vi "Remove Waveforms from ListBox.vi"(5 "Names List":bool, 7 "UI Refs":T2, 8 "error in":errorcluster, 9 "Waveform Ref LUT":variant, 10 "CD Settings in":T3 {"CD Task Dependency Ref" format="%.0x"; "CD Task Dependency" format="%.0x"}, 11 "Custom Device Ref in":T1 format="%.0x") -> (0 "error out":errorcluster, 1 "Waveform Ref LUT out":variant, 2 "CD Settings out":T3 {"CD Task Dependency Ref" format="%.0x"; "CD Task Dependency" format="%.0x"}, 3 "Custom Device Ref out":T1 format="%.0x")   [LabVIEW 2017, in "Waveform-Processing-Custom-Device System Explorer.lvlib"]
uses:
  Waveform-Processing-Custom-Device System Explorer.lvlib
  Shared/Custom Device Settings.ctl
  <vilib>/NI Veristand/Custom Device API/Custom Device Item Ref.ctl
  Types/UI Refs Ctl.ctl
  <vilib>/NI Veristand/Custom Device API/Custom Device Pointer.ctl
  NationalInstruments.VeriStand.SystemStorage
  NationalInstruments.VeriStand
  <vilib>/NI Veristand/Custom Device Tools/Custom Device Utility Library/NI VeriStand - Search for Item by Name.vi
  <userlib>/_OpenG.lib/array/array.llb/Remove Duplicates from 1D Array (String)__ogtk.vi
  <vilib>/NI VeriStand/Custom Device API/Custom Device API.lvlib
  <vilib>/NI VeriStand/Custom Device Tools/Custom Device Utility Library/Custom Device Utility Library.lvlib
  Shared/Waveform-Processing-Custom-Device Shared.lvlib
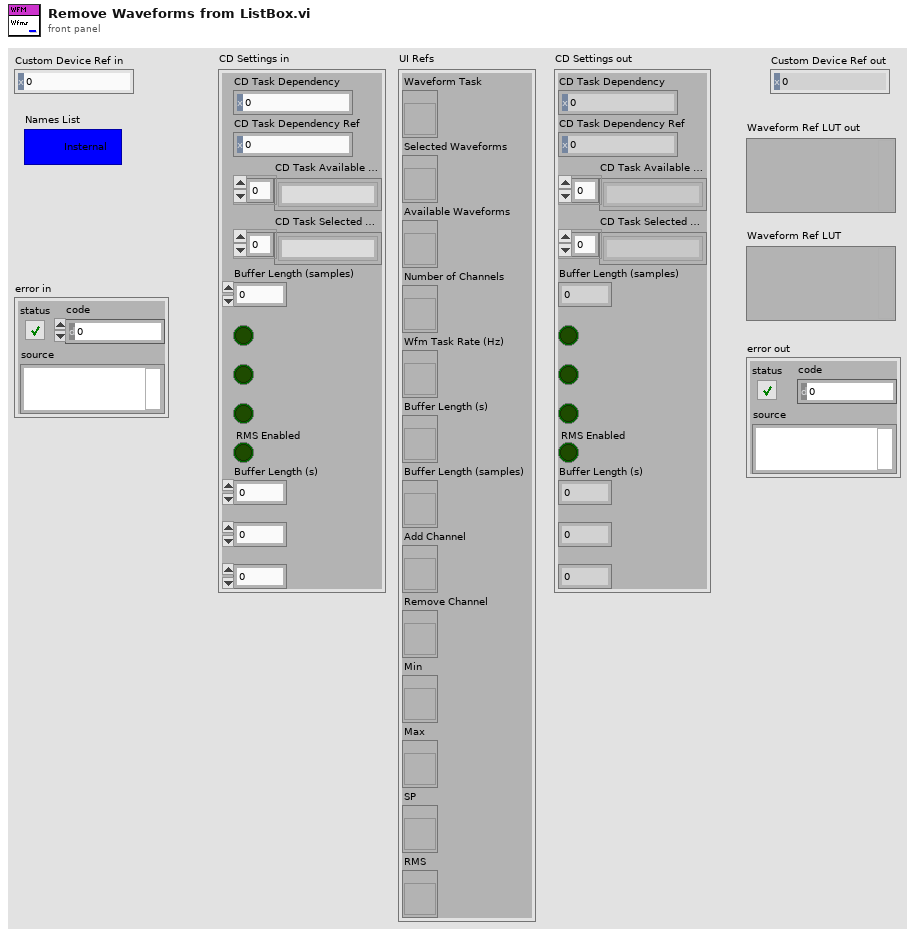
[diagram p1: front panel]
types:
  T1 = typedef "Custom Device API.lvlib/Custom Device Item Ref.ctl" = u64
  T2 = typedef "Waveform-Processing-Custom-Device Shared.lvlib/UI Refs Ctl.ctl" = cluster{"Waveform Task":refnum<vi>, "Selected Waveforms":refnum<vi>, "Available Waveforms":refnum<vi>, "Number of Channels":refnum<vi>, "Wfm Task Rate (Hz)":refnum<vi>, "Buffer Length (s)":refnum<vi>, "Buffer Length (samples)":refnum<vi>, "Add Channel":refnum<vi>, "Remove Channel":refnum<vi>, "Min":refnum<vi>, "Max":refnum<vi>, "SP":refnum<vi>, "RMS":refnum<vi>}
  T3 = typedef "Waveform-Processing-Custom-Device Shared.lvlib/Custom Device Settings.ctl" = cluster{"CD Task Dependency":T1, "CD Task Dependency Ref":T1, "CD Task Available Wfms":string[], "CD Task Selected Wfms":string[], "Buffer Length (samples)":u32, "Min Enabled":bool, "Max Enabled ":bool, "SP Enabled":bool, "RMS Enabled":bool, "Buffer Length (s)":dbl, "Task Rate":dbl, "Number of DAQ Chanels":u32}
  T4 = typedef "Custom Device API.lvlib/Custom Device Pointer.ctl" = refnum<k24>
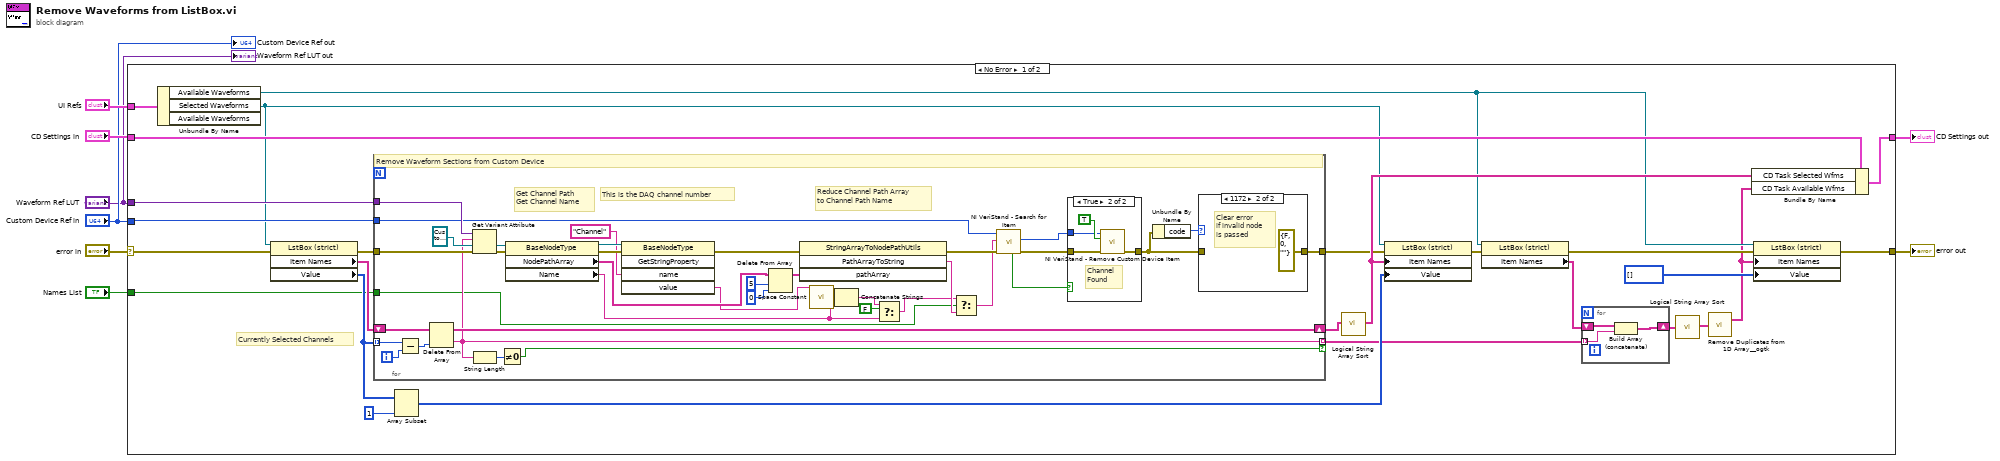
[diagram p0: block diagram]
diagram:
  n1 = case shown="No Error" "error in" {
    selector: "error in" -> [w17 w84]
    tunnel: [w30 w83] -> w8
    tunnel: "CD Settings in" -> [w29 w83]
    tunnel: [w28 w84] -> w6
    tunnel: "UI Refs" -> [w25 _]
    tunnel: "Custom Device Ref in" -> [w23 _]
    tunnel: "Waveform Ref LUT" -> [w21 _]
    tunnel: "Names List" -> [w9 _]
    frame No Error {
      # "Currently Selected Channels"
      n2 = Unbundle By Name(w25) -> ("Available Waveforms"=w24:refnum<vi>, "Selected Waveforms"=w15:refnum<vi>)  [unwired: 1 out]
      n3 = property class="LstBox (strict)"(reference=w15, error in=w17) -> (error out=w16:errorcluster, "Item Names"=w10:string[], "Value"=w14:i32[])  [unwired: 1 out]
      n4 = for {
        shift-right: [w72] -> w12
        shift-left: w10 -> [w51]
        tunnel: [w49] -> w11 mode=indexing if=w69
        tunnel: w16 -> [w64]
        tunnel: w23 -> [w57]
        tunnel: [w53] -> w22
        tunnel: w21 -> [w63]
        tunnel: w14 -> [w50] mode=indexing
        tunnel: w9 -> [w41]
        i -> [w71]
        # "This is the DAQ channel number"
        # "Reduce Channel Path Array \nto Channel Path Name"
        # "Get Channel Path\nGet Channel Name"
        # "Remove Waveform Sections from Custom Device"
        n5 = Subtract(x=w50, y=w71) -> (x-y=w70:i32)
        n6 = Delete From Array(array=w51, index=w70) -> (deleted portion=w49:string, array with subset deleted=w72:string[])  [unwired: 1 in]
        n7 = Get Variant Attribute(Variant=w63, name=w49, default value (empty Variant)=T4 refnum ("Node Pointer"), error in=w64) -> (value=w61:T4, error out=w60:errorcluster)  [unwired: 2 out]
        n8 = String Length(string=w49) -> (length=w68:i32)
        n9 = Not Equal To 0?(x=w68) -> (x != 0?=w69:bool)
        n10 = property class="BaseNodeType"(reference=w61, error in=w60) -> (reference out=w45:T4, error out=w46:errorcluster, "NodePathArray"=w47:string[], "Name"=w37:string)
        n11 = invoke class="BaseNodeType" method="GetStringProperty"(reference=w45, error in=w46, "name"="Channel") -> (error out=w35:errorcluster, "value"=w42:string)  [unwired: 2 in, 3 out]
        n12 = Delete From Array(array=w47, length=5, index=0) -> (array with subset deleted=w56:string[])  [unwired: 1 out]
        n13 = invoke class="StringArrayToNodePathUtils" method="PathArrayToString"(error in=w35, "pathArray"=w56) -> (error out=w48:errorcluster, "PathArrayToString"=w52:string)  [unwired: 2 in, 2 out]
        n14 = call <vilib>:"Space Constant.vi"() -> ("String"=w43:string)
        n15 = Concatenate Strings(w42, w43, w37) -> (w39:string)
        n16 = Select(t=w39, s=FALSE, f=w37) -> (s? t:f=w38:string)
        n17 = Select(t=w38, s=w41, f=w52) -> (s? t:f=w40:string)
        n18 = call-poly <vilib>:"NI VeriStand - Search for Item.vi"("error in"=w48, "Item Name"=w40, "Section Ref in"=w57) -> ("error out"=w67:errorcluster, "Item Ref"=w66:T1, "Found"=w65:bool)  [unwired: 5 in, 1 out]
        n19 = case shown="True" w65 {
          tunnel: [w75 w78] -> w54
          tunnel: w67 -> [w75 w77]
          tunnel: w66 -> [_ w76]
          frame False {
            # "Channel\n   NOT \nFound"
          }
          frame True {
            # "Channel\nFound"
            n20 = call <vilib>:"NI VeriStand - Remove Custom Device Item.vi"("error in (no error)"=w77, "Force Delete (F)"=TRUE, "Item Ref in"=w76) -> ("error out"=w78:errorcluster)  [unwired: 7 in, 1 out]
          }
        }
        n21 = Unbundle By Name(w54) -> ("code"=w55:i32)
        n22 = case shown="1172" w55 {
          tunnel: w54 -> [w73 _]
          tunnel: [w73 errorcluster {"status"=FALSE, "code"=0, "source"=""} ("error out")] -> w53
          frame 0, Default {
          }
          frame 1172 {
            # "Clear error\nif invalid node\nis passed"
          }
        }
      }
      n23 = Array Subset(array=w14, length=1) -> (w13:i32[])  [unwired: 1 in]
      n24 = call "Logical String Array Sort.vi"("Unsorted List"=w12) -> ("Sorted List"=w32:string[])  [unwired: 18 in]
      n25 = property on="Property Node" class="LstBox (strict)"(reference=w15, error in=w22, "Item Names"=w32, "Value"=w13) -> (error out=w26:errorcluster)  [unwired: 1 out]
      n26 = property on="Property Node" class="LstBox (strict)"(reference=w24, error in=w26) -> (error out=w27:errorcluster, "Item Names"=w31:string[])  [unwired: 1 out]
      n27 = for {
        shift-right: [w80] -> w33
        shift-left: w31 -> [w82]
        tunnel: w11 -> [w81] mode=indexing
        n28 = Build Array (concatenate)(w82, w81) -> (w80:string[])
      }
      n29 = call "Logical String Array Sort.vi"("Unsorted List"=w33) -> ("Sorted List"=w19:string[])  [unwired: 18 in]
      n30 = call-poly <userlib>:"Remove Duplicates from 1D Array__ogtk.vi"("Input Array"=w19) -> ("Output Array"=w18:string[])  [unwired: 1 out]
      n31 = Bundle By Name(cluster=w29, "CD Task Selected Wfms"=w32, "CD Task Available Wfms"=w18) -> (w30:T3)
      n32 = property on="Property Node" class="LstBox (strict)"(reference=w24, error in=w27, "Item Names"=w18, "Value"=i32[] [] ("Waveforms to Process")) -> (error out=w28:errorcluster)  [unwired: 1 out]
    }
    frame Error {
    }
  }
  "CD Settings out" <- w8
  "error out" <- w6
  "Custom Device Ref out" <- "Custom Device Ref in"
  "Waveform Ref LUT out" <- "Waveform Ref LUT"
